vi "Ch_Active_Control_Client.vi"(2 "Match":string, 3 "Activate Channels?":bool, 4 "Control on":T7) -> (0 "Editted Channels":T1[](array[typedef]) {"Duty" format="%.0b"; "D" format="%#_5g"; "C" format="%#_5g"; "B" format="%#_5g"; "A" format="%#_5g"}, 1 "No of Channels":i32)   [LabVIEW 2015]
uses:
  Sub VIs/Channel_State_Control.ctl
  Sub VIs/ADAM Controls/Ch_description_ADAM.ctl
  Sub VIs/ADAM Controls/Module_type_ADAM.ctl
  Sub VIs/ADAM Controls/Function_ADAM.ctl
  Sub VIs/ADAM Controls/Channel_State.ctl
  Sub VIs/ADAM Controls/Calib_type_ADAM.ctl
  Sub VIs/ADAM Controls/Address.ctl
  Anemometry/Anemometry Sub Vis/Globals/Preference_global.vi
panel:
  out "Iterations":i32
  in  "Ch Active Control":refnum<vi>
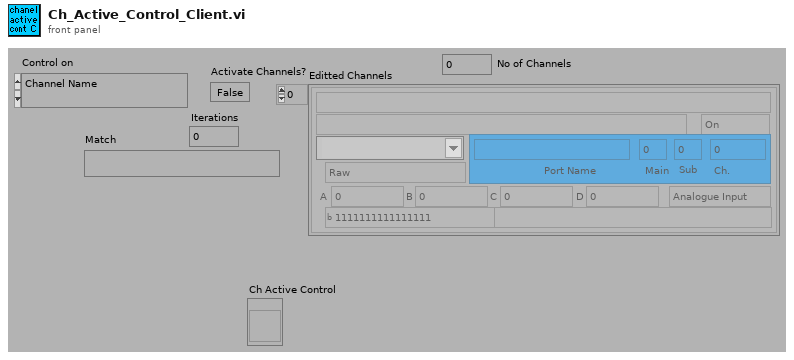
[diagram p1: front panel]
types:
  T1 = typedef "Ch_description_ADAM.ctl" = cluster{"Ch Name":string, "Type":T2, "Function":T3, "Ch State":T4, "Calibration type":T5, "A":dbl, "B":dbl, "C":dbl, "D":dbl, "Comments":string, "Address":T6, "String":string, "Duty":u16}
  T2 = typedef "Module_type_ADAM.ctl" = string
  T3 = typedef "Function_ADAM.ctl" = enum16{"Analogue Input", "Digital Input", "Event counter", "Event rate", "Analogue Output", "Digital Output", "Relay Output"}
  T4 = typedef "Channel_State.ctl" = enum16{"On", "Off", "Always On", "Always Off"}
  T5 = typedef "Calib_type_ADAM.ctl" = enum16{"Raw", "Bx + A", "Cx^2 + Bx + A", "Dx^3 + Cx^2 + Bx + A", "In Band", "Hi-Tec Q", "Hi-Tec M_dot", "Text"}
  T6 = typedef "Address.ctl" = cluster{"Main":i32, "Ch.":i32, "Sub":i32, "Port Name":string}
  T7 = typedef "Channel_State_Control.ctl" = enum16{"Channel Name", "Channel Name Starts with", "Main Address"}
  T8 = typedef "Server_Comms.ctl" = enum16{"Server Link Healthy", "Do Not Link To Server"}
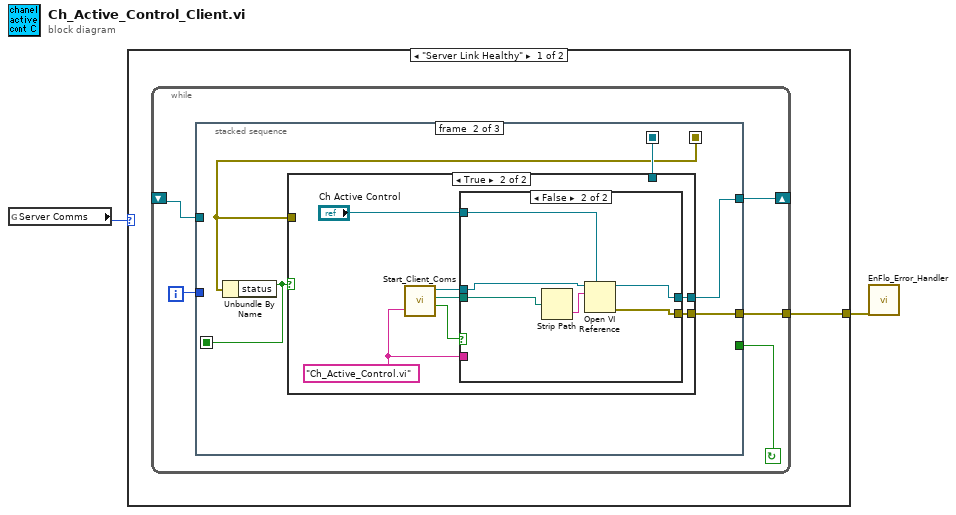
[diagram p0: block diagram]
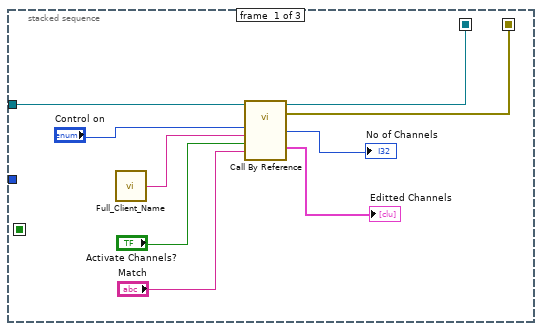
[diagram p2: hidden frame]
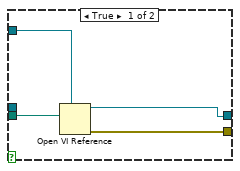
[diagram p4: hidden frame]
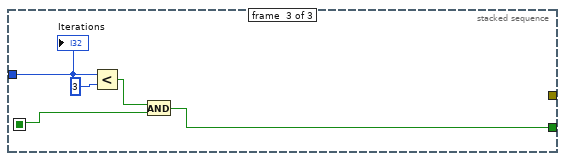
[diagram p5: hidden frame]
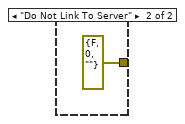
[diagram p6: hidden frame]
diagram:
  n1 = global read "Preference_global.vi" "Server Comms"() -> (w1:T8)
  n2 = case shown="\"Server Link Healthy\"" w1 {
    tunnel: [w3 errorcluster {"status"=FALSE, "code"=0, "source"=""}] -> w2
    frame "Server Link Healthy" {
      n3 = while {
        tunnel: [w4] -> w3
        shift-left: _ -> [w8]
        shift-right: [w7] -> _
        i -> [w6]
        stop <- w5 continue-if-true
        n4 = stacked-sequence {
          seq-local: [w9 _ _] -> [_ w22 _]
          seq-local: [w17 _ _] -> [_ w19 _]
          seq-local: [_ w21 _] -> [_ _ w43]
          tunnel: w8 -> [w10 _ _]
          tunnel: [_ w18 _] -> w7
          tunnel: w6 -> [_ _ w44]
          tunnel: [_ _ w42] -> w5
          tunnel: [_ w20 _] -> w4
          frame #0 {
            n5 = call "Full_Client_Name.vi"() -> ("Client Name"=w16:string)
            n6 = call-by-ref "?"(reference=w10, "Match"="Match", "Activate Channels?"="Activate Channels?", "Client Name"=w16, "Control on"="Control on") -> (reference out=w9:refnum<vi>, error out=w17:errorcluster, "Editted Channels"=→"Editted Channels":T1[], "No of Channels"=→"No of Channels":i32)  [unwired: 1 in]
          }
          frame #1 {
            n7 = Unbundle By Name(w19) -> ("status"=w21:bool)
            n8 = case shown="True" w21 {
              tunnel: w22 -> [w23 _]
              tunnel: [w24 w28] -> w20
              tunnel: w19 -> [w24 _]
              tunnel: [w23 w27] -> w18
              frame False {
              }
              frame True {
                w26 = "Ch_Active_Control.vi"
                n9 = call "Start_Client_Coms.vi"("VI name to run on server"=w26) -> ("LabVIEW application reference"=w31:refnum<vi>, "Checked VI name"=w29:path, "Local Call"=w30:bool)  [unwired: 1 in, 1 out]
                n10 = case shown="False" w30 {
                  tunnel: w29 -> [w35 w40]
                  tunnel: w31 -> [_ w39]
                  tunnel: [w34 w36] -> w28
                  tunnel: [w33 w37] -> w27
                  tunnel: w26 -> [_ _]
                  tunnel: "Ch Active Control" -> [w32 w38]
                  frame True {
                    n11 = Open VI Reference(type specifier VI Refnum (for type only)=w32, vi path=w35) -> (vi reference=w33:refnum<vi>, error out=w34:errorcluster)  [unwired: 1 in, 3 out]
                  }
                  frame False {
                    n12 = Strip Path(path=w40) -> (name=w41:string)  [unwired: 1 out]
                    n13 = Open VI Reference(type specifier VI Refnum (for type only)=w38, application reference (local)=w39, vi path=w41) -> (vi reference=w37:refnum<vi>, error out=w36:errorcluster)  [unwired: 1 in, 2 out]
                  }
                }
              }
            }
          }
          frame #2 {
            n14 = Less?(x=w44, y=3) -> (x < y?=w46:bool)
            n15 = And(x=w46, y=w43) -> (x .and. y?=w42:bool)
            "Iterations" <- w44
          }
        }
      }
    }
    frame "Do Not Link To Server" {
    }
  }
  n16 = call "EnFlo_Error_Handler.vi"("error in (no error)"=w2) -> ()  [unwired: 2 in, 3 out]
